vi "Close Connection.vi"(8 "error in (no error)":errorcluster, 11 "BLE context in":refnum<class "BLE context.lvclass">) -> (0 "error out":errorcluster, 3 "BLE context out":refnum<class "BLE context.lvclass">)   [LabVIEW 2015, in "BLE context.lvclass"]
uses:
  BLE context.lvclass
  BLE context.lvclass/BLE context.ctl
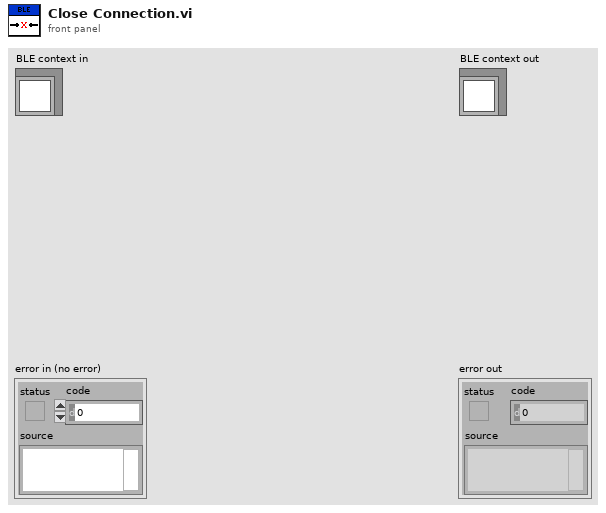
[diagram p1: front panel]
types:
  T1 = typedef "connection_status_bundle.ctl" = cluster{"MAC Address":string, "cnx handle":u8, "cnx flags":u8, "Address Type":T2, "Connection Interval (ms)":u16, "Timeout(ms)":u16, "Latency":u16, "bonding handle":u8}
  T2 = typedef "address_type.ctl" = u8
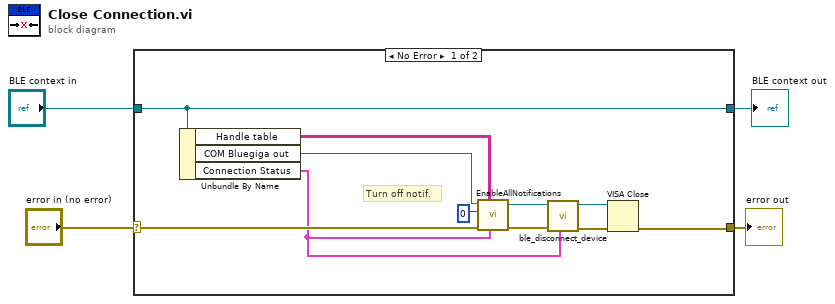
[diagram p0: block diagram]
diagram:
  n1 = case shown="No Error" "error in (no error)" {
    selector: "error in (no error)" -> [w9 w17]
    tunnel: [w5 w17] -> w3
    tunnel: [w10 w16] -> w1
    tunnel: "BLE context in" -> [w10 w16]
    frame No Error {
      # "Turn off notif."
      n2 = Unbundle By Name(w10) -> ("Handle table"=w7:string[][], "COM Bluegiga out"=w8:refnum<visa-resource-name>, "Connection Status"=w6:T1)
      n3 = call "EnableAllNotifications.vi"("Connection Status"=w6, "Handle table"=w7, "error in"=w9, "1 or 0"=u16 0, "COM Bluegiga in"=w8) -> ("error out"=w12:errorcluster, "COM Bluegiga out"=w11:refnum<visa-resource-name>)  [unwired: 5 in]
      n4 = call <vilib>:"ble_disconnect_device.vi"("Connection Status"=w6, "error in (no error)"=w12, "COM Bluegiga in"=w11) -> ("error out"=w14:errorcluster, "COM Bluegiga out"=w15:refnum<visa-resource-name>)  [unwired: 7 in]
      n5 = VISA Close(VISA resource name=w15, error in (no error)=w14) -> (error out=w5:errorcluster)
    }
    frame Error {
    }
  }
  "error out" <- w3
  "BLE context out" <- w1
